vi "_DownloadPackageFromNevstopFTP.vi"(8 "error in (no error)":errorcluster, 10 "RemoteDirectory":string="/nevstop-lab/LabVIEW-Tag-Container", 11 "ftp":T1={"address"="vipm.nevstop.top", "remote port (21)"=1986, "userName"="", "passWord"=""}) -> (0 "error out":errorcluster, 2 "candidates":T2[](array[typedef]), 3 "localdir":path, 4 "Array":string[](array[string]))   [LabVIEW 2014]
uses:
  _support/FTP Toolkit/FTP Class/controls/Dir-File Info.ctl
  _support/FTP Toolkit/FTP Class/controls/Dir-File Type.ctl
  _support/FTP Toolkit/FTP Class/FTP.lvclass
  <userlib>/_OpenG.lib/array/array.llb/Sort 1D Array (String)__ogtk.vi
  <userlib>/_OpenG.lib/array/array.llb/Reorder 1D Array2 (Variant)__ogtk.vi
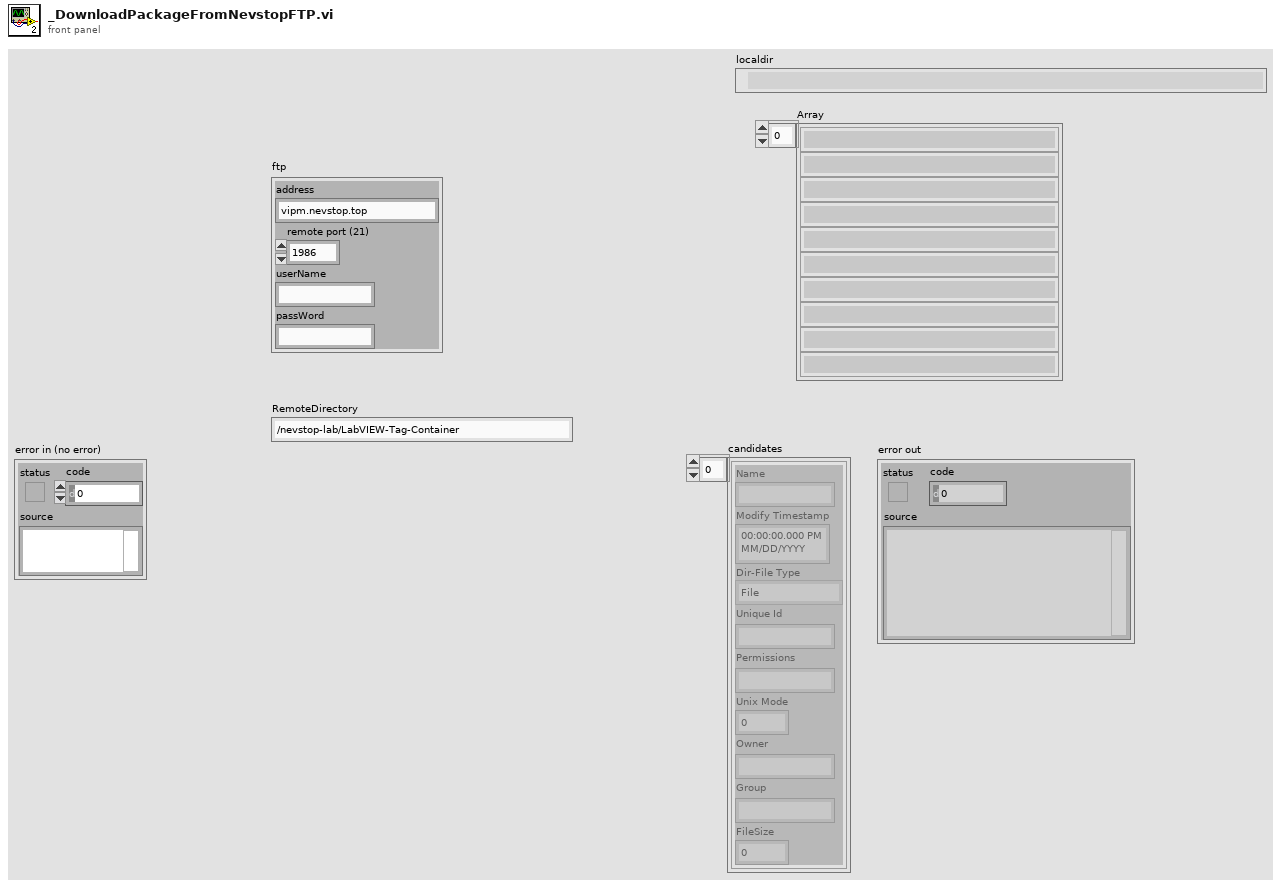
[diagram p1: front panel]
types:
  T1 = cluster{"address":string, "remote port (21)":u16, "userName":string, "passWord":string}
  T2 = typedef "FTP.lvlib/FTP.lvclass/Dir-File Info.ctl" = cluster{"Name":string, "Modify Timestamp":timestamp, "Dir-File Type":T3, "Unique Id":string, "Permissions":string, "Unix Mode":u16, "Owner":string, "Group":string, "FileSize":i64}
  T3 = typedef "FTP.lvlib/FTP.lvclass/Dir-File Type.ctl" = enum16{"File", "Listed Directory", "Parent Directory", "Directory", "Unknown"}
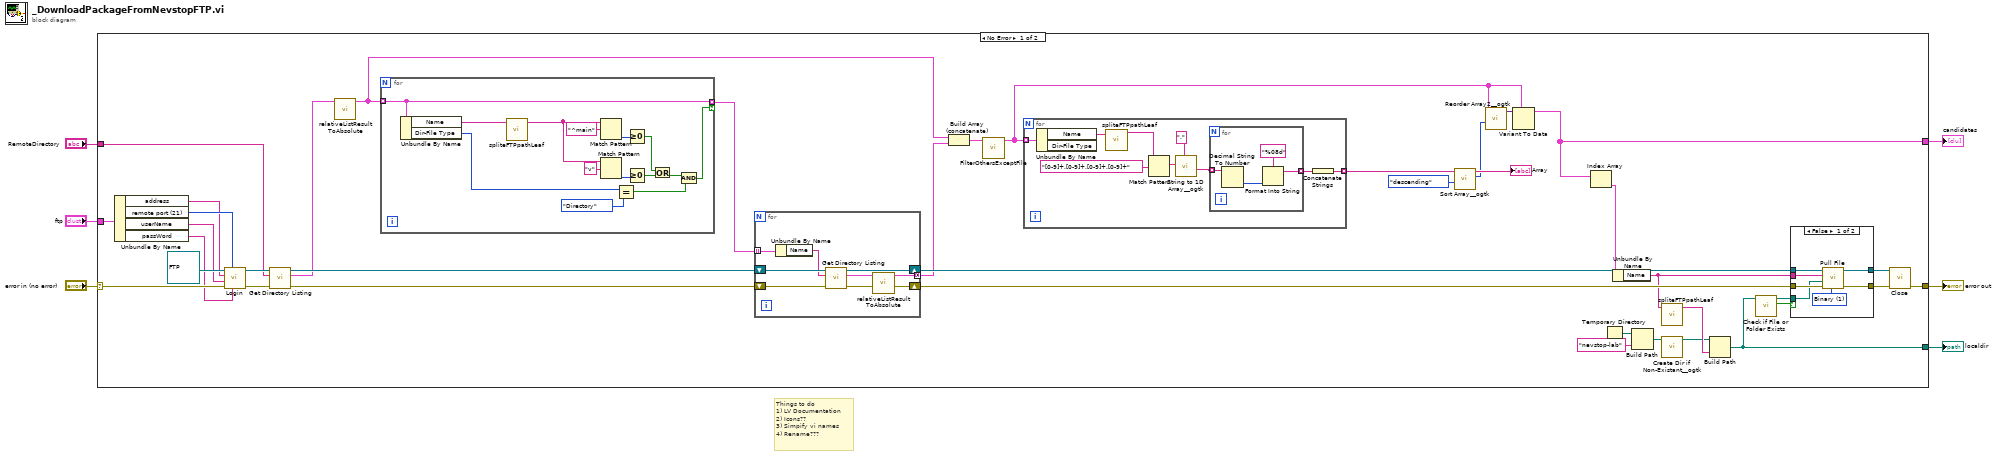
[diagram p0: block diagram]
diagram:
  # "Things to do\n1) LV Documentation\n2) Icons??\n3) Simpify vi names\n4) Rename???"
  n1 = case shown="No Error" "error in (no error)" {
    selector: "error in (no error)" -> [w43 w90]
    tunnel: [w45 w90] -> w5
    tunnel: [w7 _] -> w4
    tunnel: [w17 _] -> w3
    tunnel: "ftp" -> [w15 _]
    tunnel: "RemoteDirectory" -> [w10 _]
    frame No Error {
      n2 = Unbundle By Name(w15) -> ("address"=w13:string, "remote port (21)"=w14:u16, "userName"=w12:string, "passWord"=w11:string)
      n3 = call "Login.vi"("passWord"=w11, "remote port (21)"=w14, "error in (no error)"=w43, "userName"=w12, "address"=w13, "FTP in"=refnum<class "FTP.lvclass"> refnum) -> ("error out"=w42:errorcluster, "FTP out"=w44:refnum<class "FTP.lvclass">)  [unwired: 4 in]
      n4 = call "Get Directory Listing.vi"("error in (no error)"=w42, "RemoteDirectory"=w10, "FTP in"=w44) -> ("error out"=w40:errorcluster, "Dir-File Info Array"=w34:T2[], "FTP out"=w41:refnum<class "FTP.lvclass">)  [unwired: 6 in]
      n5 = call "relativeListResultToAbsolute.vi"("Dir-File Info Array"=w34) -> ("Array"=w33:T2[])  [unwired: 10 in]
      n6 = for {
        tunnel: w33 -> [w83] mode=indexing
        tunnel: [w83] -> w39 mode=indexing if=w82
        n7 = Unbundle By Name(w83) -> ("Name"=w77:string, "Dir-File Type"=w88:T3)
        n8 = call "spliteFTPpathLeaf.vi"("Name"=w77) -> ("String"=w76:string)  [unwired: 10 in]
        n9 = Match Pattern(string=w76, regular expression="^main") -> (offset past match=w81:i32)  [unwired: 1 in, 3 out]
        n10 = Match Pattern(string=w76, regular expression="v") -> (offset past match=w86:i32)  [unwired: 1 in, 3 out]
        n11 = Equal?(x=w88, y=Dir-File_Type."Directory") -> (x = y?=w84:bool)
        n12 = Greater Or Equal To 0?(x=w81) -> (x >= 0?=w78:bool)
        n13 = Greater Or Equal To 0?(x=w86) -> (x >= 0?=w85:bool)
        n14 = Or(x=w78, y=w85) -> (x .or. y?=w79:bool)
        n15 = And(x=w79, y=w84) -> (x .and. y?=w82:bool)
      }
      n16 = for {
        tunnel: w39 -> [w73] mode=indexing
        tunnel: [w68] -> w36 mode=concatenating
        shift-right: [w70] -> w37
        shift-left: w41 -> [w75]
        shift-right: [w71] -> w38
        shift-left: w40 -> [w74]
        n17 = Unbundle By Name(w73) -> ("Name"=w72:string)
        n18 = call "Get Directory Listing.vi"("error in (no error)"=w74, "RemoteDirectory"=w72, "FTP in"=w75) -> ("error out"=w71:errorcluster, "Dir-File Info Array"=w69:T2[], "FTP out"=w70:refnum<class "FTP.lvclass">)  [unwired: 6 in]
        n19 = call "relativeListResultToAbsolute.vi"("Dir-File Info Array"=w69) -> ("Array"=w68:T2[])  [unwired: 10 in]
      }
      n20 = Build Array (concatenate)(w33, w36) -> (w35:T2[])
      n21 = call "FilterOthersExceptFile.vi"("Array in"=w35) -> ("Array out"=w27:T2[])  [unwired: 10 in]
      n22 = for {
        tunnel: w27 -> [w63] mode=indexing
        tunnel: [w55] -> w31 mode=indexing
        n23 = Unbundle By Name(w63) -> ("Name"=w62:string)  [unwired: 1 out]
        n24 = call "spliteFTPpathLeaf.vi"("Name"=w62) -> ("String"=w60:string)  [unwired: 10 in]
        n25 = Match Pattern(string=w60, regular expression="[0-9]+.[0-9]+.[0-9]+.[0-9]+") -> (match substring=w59:string)  [unwired: 1 in, 3 out]
        n26 = call <userlib>:"String to 1D Array__ogtk.vi"("delimiter (Tab)"=".", "string"=w59) -> ("Array of Strings"=w57:string[])  [unwired: 9 in]
        n27 = for {
          tunnel: w57 -> [w67] mode=indexing
          tunnel: [w65] -> w56 mode=indexing
          n28 = Decimal String To Number(string=w67) -> (number=w64:i32)  [unwired: 2 in, 1 out]
          n29 = Format Into String(format string="%08d", w64) -> (resulting string=w65:string)  [unwired: 2 in, 1 out]
        }
        n30 = Concatenate Strings(w56) -> (w55:string)
      }
      n31 = call-poly <userlib>:"Sort Array__ogtk.vi"("Order"=enum16{"ascending", "descending"}."descending", "Array in"=w31) -> ("Sorted Pointers"=w29:i32[], "Sorted Array out"=→"Array":string[])  [unwired: 8 in]
      n32 = call-poly <userlib>:"Reorder Array2__ogtk.vi"("indices"=w29, "array"=w27) -> ("reordered array"=w28:variant[])  [unwired: 9 in]
      n33 = Variant To Data(type=w27, Variant=w28) -> (data=w17:T2[])  [unwired: 1 in, 1 out]
      n34 = Index Array(array=w17) -> (element=w24:T2)  [unwired: 1 in]
      n35 = Temporary Directory() -> (w23:path)
      n36 = Unbundle By Name(w24) -> ("Name"=w20:string)
      n37 = Build Path(base path=w23, name or relative path="nevstop-lab") -> (appended path=w22:path)
      n38 = call "spliteFTPpathLeaf.vi"("Name"=w20) -> ("String"=w19:string)  [unwired: 10 in]
      n39 = call <userlib>:"Create Dir if Non-Existant__ogtk.vi"("Directory Path"=w22) -> ("dup Directory Path"=w18:path)  [unwired: 8 in, 2 out]
      n40 = Build Path(base path=w18, name or relative path=w19) -> (appended path=w7:path)
      n41 = call <vilib>:"Check if File or Folder Exists.vi"("path"=w7) -> ("file or folder exists?"=w8:bool, "dup path"=w9:path)  [unwired: 8 in, 1 out]
      n42 = case shown="False" w8 {
        tunnel: w38 -> [w51 w53]
        tunnel: w37 -> [w50 w54]
        tunnel: [w49 w54] -> w26
        tunnel: [w48 w53] -> w25
        tunnel: w20 -> [w47 _]
        tunnel: w9 -> [w46 _]
        frame False {
          w52 = u16 1 items=["ASCII", "Binary"] ("Type")
          n43 = call "Pull File.vi"("Type (Binary)"=w52, "error in (no error)"=w51, "Local FilePath"=w46, "FileName"=w47, "FTP in"=w50) -> ("error out"=w48:errorcluster, "FTP out"=w49:refnum<class "FTP.lvclass">)  [unwired: 5 in]
        }
        frame True {
        }
      }
      n44 = call "Close.vi"("error in (no error)"=w25, "FTP in"=w26) -> ("error out"=w45:errorcluster)  [unwired: 9 in]
    }
    frame Error {
    }
  }
  "error out" <- w5
  "localdir" <- w4
  "candidates" <- w3
